vi "Phase Noise Display Setup.vi"(6 "Display Line Level (-2.5 Amplitude Units)":dbl=-2.5, 7 "Enable Display Line (Enable)":bool=TRUE, 8 "error in (no error)":errorcluster, 9 "Display Marker Table (T: Enable)":bool=TRUE, 10 "Display Decade Table (T: Enable)":bool=TRUE, 11 "VISA resource name":refnum<visa-resource-name>) -> (0 "error out":errorcluster, 3 "VISA resource name out":refnum<visa-resource-name>)   [LabVIEW 2014, in "Agilent ESA PSA Series.lvlib"]
doc: "Sets the analyzer phase noise display settings.\n\n<B>Note:</B>\n\nThis VI is only valid in Phase Noise personality. Use <B>Switch Personality</B> VI to switch to Phase Noise before calling this VI."
uses:
  Agilent ESA PSA Series.lvlib
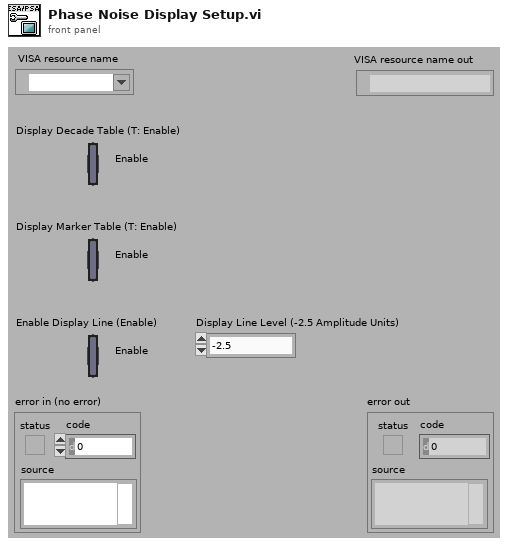
[diagram p1: front panel]
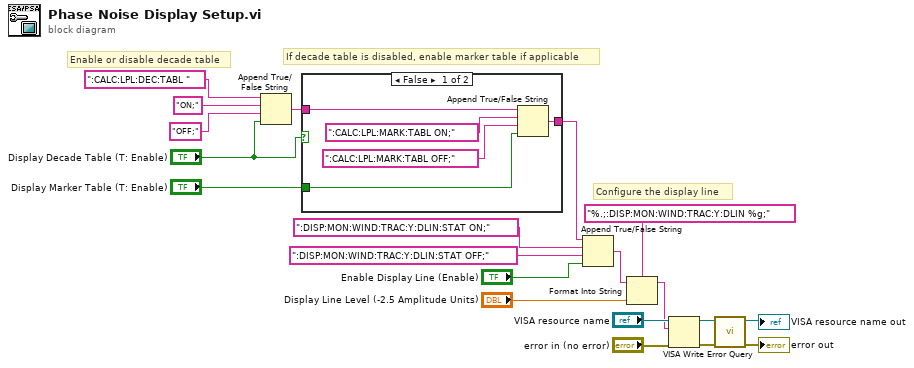
[diagram p0: block diagram]
diagram:
  # "Configure the display line"
  # "If decade table is disabled, enable marker table if applicable"
  # "Enable or disable decade table"
  n1 = Append True/False String(1:"Display Decade Table (T: Enable)", 2:"OFF;" ("true string"), 3:"ON;" ("true string"), 4:":CALC:LPL:DEC:TABL " ("string (\"\")")) -> (0:w2:string)
  n2 = case shown="False" "Display Decade Table (T: Enable)" {
    tunnel: [w23 w26] -> w4
    tunnel: "Display Marker Table (T: Enable)" -> [w22 _]
    tunnel: w2 -> [w21 w26]
    frame False {
      n3 = Append True/False String(1:w22, 2:":CALC:LPL:MARK:TABL OFF;" ("false string"), 3:":CALC:LPL:MARK:TABL ON;" ("true string"), 4:w21) -> (0:w23:string)
    }
    frame True {
    }
  }
  n4 = Append True/False String(1:"Enable Display Line (Enable)", 2:":DISP:MON:WIND:TRAC:Y:DLIN:STAT OFF;" ("false string"), 3:":DISP:MON:WIND:TRAC:Y:DLIN:STAT ON;" ("true string"), 4:w4) -> (0:w7:string)
  n5 = Format Into String(format string="%.;:DISP:MON:WIND:TRAC:Y:DLIN %g;", initial string=w7, "Display Line Level (-2.5 Amplitude Units)") -> (resulting string=w5:string)  [unwired: 1 in, 1 out]
  n6 = VISA Write(VISA resource name="VISA resource name", write buffer=w5, error in (no error)="error in (no error)") -> (VISA resource name out=w18:refnum<visa-resource-name>, error out=w17:errorcluster)  [unwired: 1 out]
  n7 = call "Error Query.vi"("error in (no error)"=w17, "VISA resource name"=w18) -> ("error out"=→"error out":errorcluster, "VISA resource name out"=→"VISA resource name out":refnum<visa-resource-name>)  [unwired: 6 in, 2 out]
